vi "PPFS_TRAJ_ABS_ODOM_EXECUTE.vi"(6 "Pass_Through_Time":dbl=-1.0 format="%33.4f", 8 "error in (no error)":errorcluster) -> (0 "error out":errorcluster)   [LabVIEW 2019]
uses:
  <vilib>/Rock Robotics/WPI/ThirdParty/JAS_Junk/TrajLib/Rotation2d_Plus.vi
  <vilib>/Rock Robotics/WPI/ThirdParty/JAS_Junk/TrajLib/Twist2d_Create.vi
  <vilib>/Rock Robotics/WPI/ThirdParty/JAS_Junk/TrajLib/Rotation2d_Minus.vi
  <vilib>/Rock Robotics/WPI/ThirdParty/JAS_Junk/TrajLib/Pose2d_getTranslation.vi
  <vilib>/Rock Robotics/WPI/ThirdParty/JAS_Junk/TrajLib/Pose2d_New_TRRO.vi
  <vilib>/Rock Robotics/WPI/ThirdParty/JAS_Junk/TrajLib/VI/SwerveModulePosition_Get.vi
  <vilib>/Rock Robotics/WPI/ThirdParty/JAS_Junk/TrajLib/VI/SwerveModulePosition_New.vi
  <vilib>/Rock Robotics/WPI/ThirdParty/JAS_Junk/TrajLib/Twist2d_GetAll.vi
  <vilib>/Rock Robotics/WPI/ThirdParty/JAS_Junk/TrajLib/VI/Util_GetTime_U32.vi
  <vilib>/Rock Robotics/WPI/ThirdParty/JAS_Junk/TrajLib/Rotation2d_RotateBy.vi
  <vilib>/Rock Robotics/WPI/ThirdParty/JAS_Junk/TrajLib/Rotation2d_UnaryMinus.vi
  <vilib>/Rock Robotics/WPI/ThirdParty/JAS_Junk/TrajLib/Rotation2d_CreateXY.vi
  <vilib>/Rock Robotics/WPI/ThirdParty/JAS_Junk/TrajLib/Util_CalcDist.vi
  Swerve_Drive_System/PPFS_DRIVE_GLOBALS.vi
  PPFS_TRAJECTORY_GLOBALS.vi
  <vilib>/Rock Robotics/WPI/ThirdParty/JAS_Junk/TrajLib/VI/SwerveKinematics_ToTwist2dX.vi
  <vilib>/Rock Robotics/WPI/ThirdParty/JAS_Junk/TrajLib/Pose2d_Exp.vi
  <vilib>/Rock Robotics/WPI/ThirdParty/JAS_Junk/TrajLib/VI/Util_GetTime_U64.vi
  <vilib>/Rock Robotics/WPI/ThirdParty/JAS_Junk/TrajLib/Trajectory_Library.lvlib
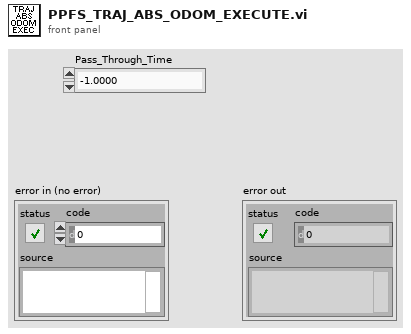
[diagram p1: front panel]
types:
  T1 = typedef "Trajectory_Library.lvlib/SWERVE_DRIVE_MODULE_POSITION.ctl" = cluster{"Distance":dbl, "Angle":T2, "P":bool}
  T2 = typedef "Trajectory_Library.lvlib/ROTATION2D.ctl" = cluster{"VALUE":dbl, "COS":dbl, "SIN":dbl}
  T3 = typedef "Trajectory_Library.lvlib/SWERVE_DRIVE_KINEMATICS.ctl" = cluster{"NumModules":i32, "InverseKinematics":T4, "ForwardKinematics":T4, "Modules":T5[], "PrevCoR":T5, "SavedModuleStates":T6[]}
  T4 = typedef "NI_Matrix.lvlib/RealMatrix.ctl" = dbl[][]
  T5 = typedef "Trajectory_Library.lvlib/TRANSLATION2D.ctl" = cluster{"X":dbl, "Y":dbl}
  T6 = typedef "Trajectory_Library.lvlib/SWERVE_DRIVE_MODULE_STATE.ctl" = cluster{"Speed":dbl, "Angle":T2}
  T7 = typedef "Trajectory_Library.lvlib/SWERVE_DRIVE_ODOMETRY.ctl" = cluster{"POSE":T8, "GyroOffset":T2, "PreviousAngle":T2, "PrevModulePositions":T1[], "NumModules":i32}
  T8 = typedef "Trajectory_Library.lvlib/POSE2D.ctl" = cluster{"TRANSLATION":T5, "ROTATION":T2}
  T9 = typedef "Trajectory_Library.lvlib/SWERVE_DRIVE_POSE_EST2_CONFIG.ctl" = cluster{"Wheel_Locations M":T5[], "Odom X std dev M":dbl, "Odom Y std dev M":dbl, "Odom Heading std dev Rad":dbl, "Vision X std dev M":dbl, "Vision Y std dev M":dbl, "Vision Heading std dev Rad":dbl}
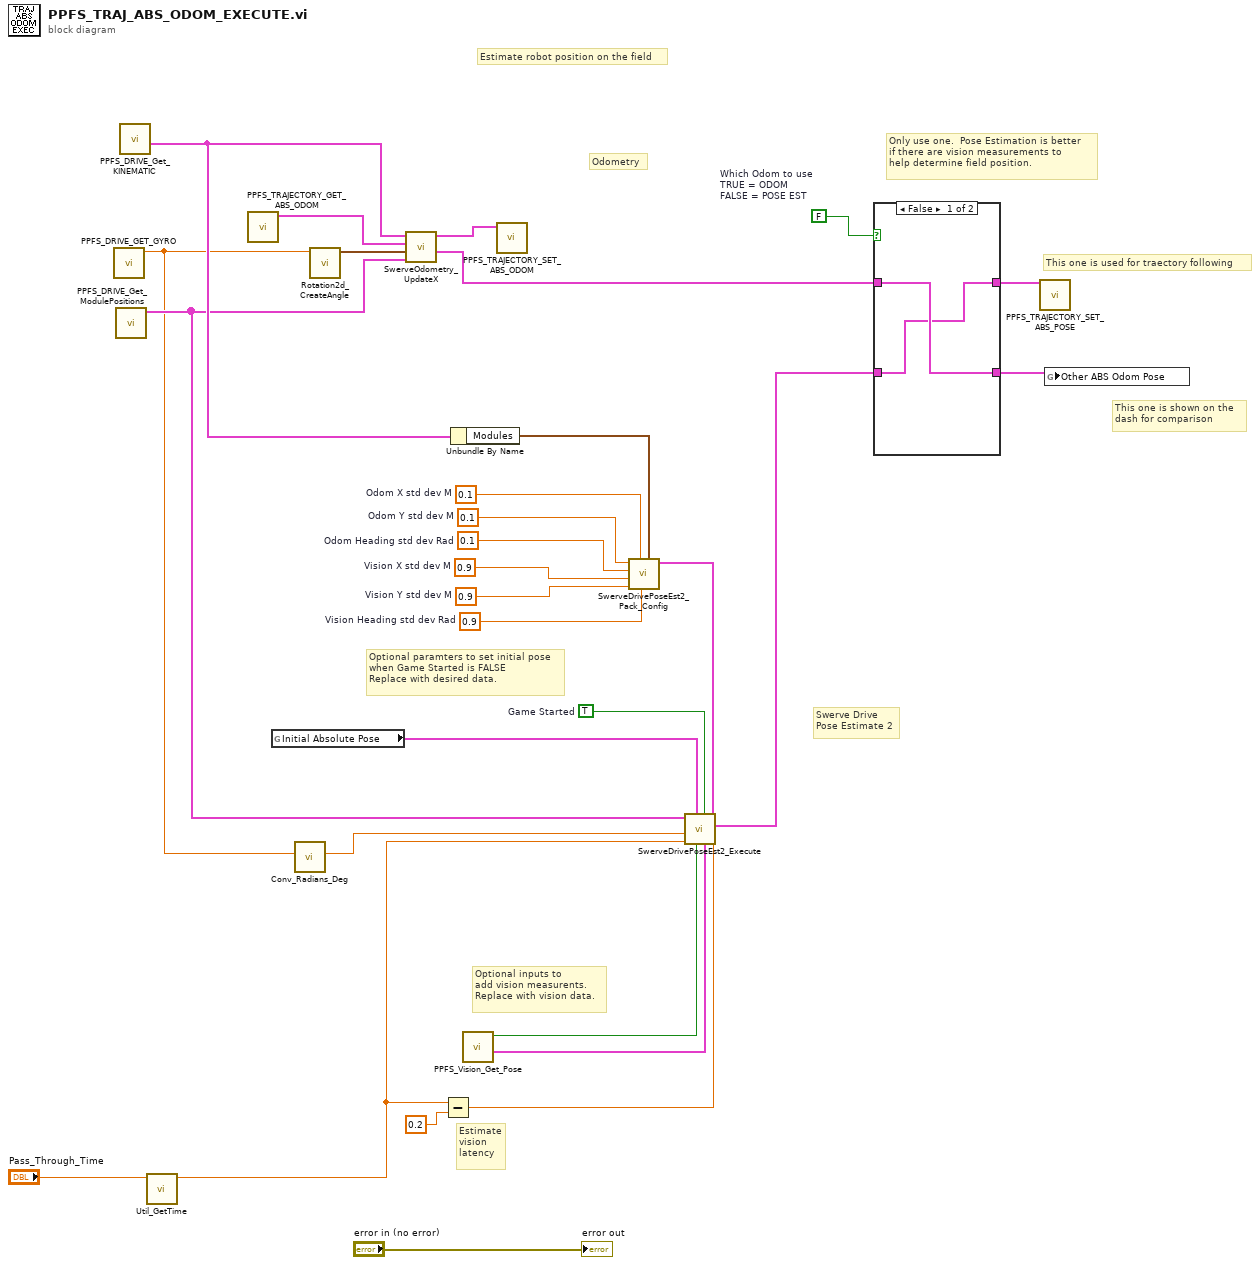
[diagram p0: block diagram]
diagram:
  w6 = FALSE  # Which Odom to use TRUE = ODOM FALSE = POSE EST
  w16 = TRUE  # Game Started
  w17 = 0.1  # Odom Y std dev M
  w18 = 0.1  # Odom Heading std dev Rad
  w19 = 0.9  # Vision X std dev M
  w20 = 0.9  # Vision Y std dev M
  w21 = 0.1  # Odom X std dev M
  w22 = 0.9  # Vision Heading std dev Rad
  # "Estimate\nvision \nlatency"
  # "This one is shown on the\ndash for comparison"
  # "This one is used for traectory following"
  # "Only use one.  Pose Estimation is better\nif there are vision measurements to\nhelp determine field position."
  # "Optional inputs to\nadd vision measurents.\nReplace with vision data."
  # "Optional paramters to set initial pose\nwhen Game Started is FALSE\nReplace with desired data."
  # "Swerve Drive \nPose Estimate 2"
  # "Odometry"
  # "Estimate robot position on the field"
  n1 = call "PPFS_DRIVE_GET_GYRO.vi"() -> ("Gyro Heading Radians"=w12:dbl)  [unwired: 11 in]
  n2 = call "PPFS_DRIVE_Get_ModulePositions.vi"() -> ("Swerve Module Positions"=w27:T1[])  [unwired: 11 in]
  n3 = call "PPFS_DRIVE_Get_KINEMATIC.vi"() -> ("out SWERVE_DRIVE_KINEMATICS"=w28:T3)  [unwired: 11 in]
  n4 = call <vilib>:"Util_GetTime.vi"("Pass_Through_Time"="Pass_Through_Time") -> ("FPGA_Time_Seconds"=w5:dbl)  [unwired: 8 in, 2 out]
  n5 = call "PPFS_TRAJECTORY_GET_ABS_ODOM.vi"() -> ("Absolue Odometry"=w24:T7)  [unwired: 11 in]
  n6 = global read "PPFS_TRAJECTORY_GLOBALS.vi" "Initial Absolute Pose"() -> (w13:T8)
  n7 = call <vilib>:"Conv_Radians_Deg.vi"("Radians"=w12) -> ("Degrees"=w11:dbl)  [unwired: 10 in]
  n8 = call <vilib>:"Rotation2d_CreateAngle.vi"("Angle"=w12) -> ("ROTATION"=w25:T2)  [unwired: 10 in]
  n9 = call <vilib>:"SwerveOdometry_UpdateX.vi"("module Positions"=w27, "gyroAngle"=w25, "in SWERVE_DRIVE_ODOMETRY"=w24, "SWERVE_DRIVE_KINEMATICS"=w28) -> ("robot POSE"=w10:T8, "out SWERVE_DRIVE_ODOMETRY"=w23:T7)  [unwired: 5 in, 1 out]
  n10 = Subtract(x=w5, y=0.2) -> (x-y=w3:dbl)
  n11 = Unbundle By Name(w28) -> ("Modules"=w14:T5[])
  n12 = call "PPFS_Vision_Get_Pose.vi"() -> ("Vison Pose"=w1:T8, "Have Vision Pose"=w2:bool)  [unwired: 10 in]
  n13 = call "PPFS_TRAJECTORY_SET_ABS_ODOM.vi"("Absolue Odometry"=w23) -> ()  [unwired: 11 in]
  n14 = call <vilib>:"SwerveDrivePoseEst2_Pack_Config.vi"("Wheel_Locations M"=w14, "Vision Heading std dev Rad"=w22, "Odom X std dev M"=w21, "Vision Y std dev M"=w20, "Vision X std dev M"=w19, "Odom Heading std dev Rad"=w18, "Odom Y std dev M"=w17) -> ("SwervePoseEst2Config"=w15:T9)  [unwired: 4 in]
  n15 = call <vilib>:"SwerveDrivePoseEst2_Execute.vi"("Vision TImeStamp_Seconds"=w3, "SwervePoseEst2Config"=w15, "visionRobotPose"=w1, "Game Started"=w16, "Add Vision Meas"=w2, "InitialPose"=w13, "Pass Through Time"=w5, "Gyro Degrees"=w11, "Module Positions"=w27) -> ("Estimated Pose"=w8:T8)  [unwired: 1 in, 1 out]
  n16 = case shown="False" w6 {
    tunnel: w10 -> [w31 w33]
    tunnel: [w30 w33] -> w9
    tunnel: w8 -> [w30 w32]
    tunnel: [w31 w32] -> w7
    frame False {
    }
    frame True {
    }
  }
  n17 = call "PPFS_TRAJECTORY_SET_ABS_POSE.vi"("Absolute Odometry Pose"=w9) -> ()  [unwired: 11 in]
  n18 = global write "PPFS_TRAJECTORY_GLOBALS.vi" "Other ABS Odom Pose"(w7) -> ()
  "error out" <- "error in (no error)"
